vi "Control_Rack_Controler.vi"(0 "Times":dbl[](array[numeric]), 1 "Voltages Toroidal (Keep below |10|)":dbl[](array[numeric]), 2 "Voltages Helical (Keep below |10|)":dbl[](array[numeric]), 3 "error out":errorcluster, 4 "Data out 2":T2) -> (5 "error out 2":errorcluster, 6 "Data out":T2)   [LabVIEW 2017]
uses:
  Type_Defs/Data.ctl
  Type_Defs/Diagnostics.ctl
  Type_Defs/Systems.ctl
  <vilib>/DAQmx/write.llb/DAQmx Write (Analog DBL 1Chan 1Samp).vi
  <vilib>/DAQmx/create/channels.llb/DAQmx Create Channel (AO-Voltage-Basic).vi
  <vilib>/DAQmx/miscellaneous.llb/DAQmx Fill In Error Info.vi
  <vilib>/express/express shared/transition.llb/Dynamic To Waveform Array.vi
  <vilib>/express/express signal manip/GetorSetDDTAttributes/Set DDT Attributes/SetT0.vi
  <vilib>/express/express shared/transition.llb/Waveform Array To Dynamic.vi
  <vilib>/express/express signal manip/GetorSetDDTAttributes/Set DDT Attributes/Set DDT Properties.xnode
panel:
  out "Experiment State":T1(ring)
  out "Experiment Purpose":string
  out "Start Time":timestamp
  out "Experiment Number":i32
  out "Operator":string
  out "Running":bool
  out "hel_cur":dynamicdata(graph) caption="Helix Current Feedback"
  out "hel_vol":dynamicdata(graph) caption="Helix Voltage Feedback"
  out "hel_cur_set":dynamicdata(graph) caption="Helix Limited Current Set Point"
  out "torr_cur_set":dynamicdata(graph) caption="Torroidal Limited Current Set Point"
  out "torr_vol":dynamicdata(graph) caption="Torroidal Voltage Feedback"
  out "torr_cur":dynamicdata(graph) caption="Torroidal Current Feedback"
  out "Voltage Toroidal":dbl
  out "Time":dbl
  out "Voltage Helical":dbl
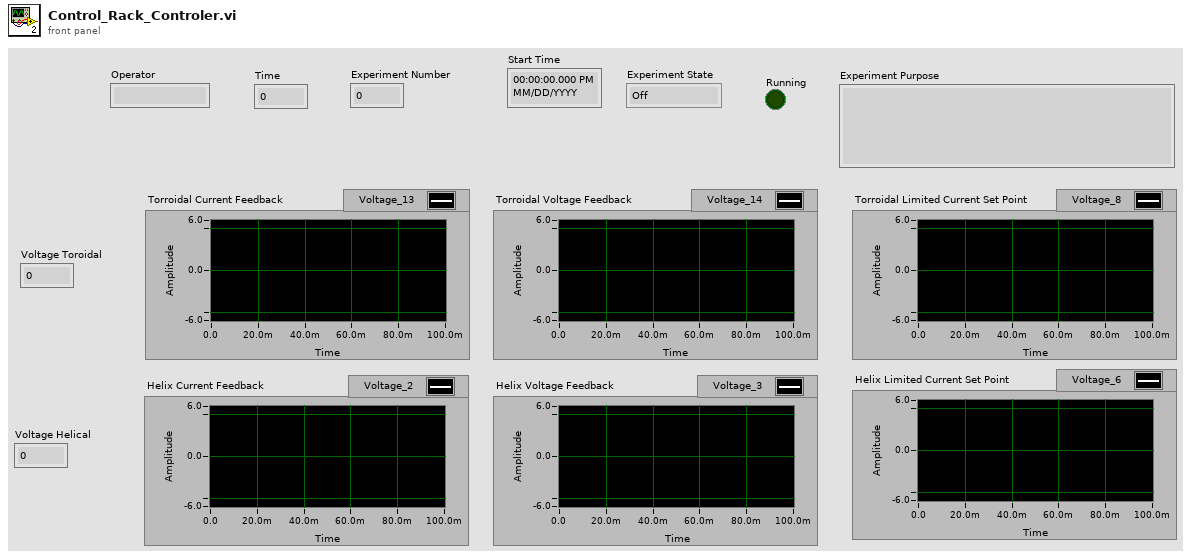
[diagram p1: front panel]
types:
  T1 = enum16{"Off", "Setting Up", "Ready", "In Progress", "Shutting Down"}
  T2 = typedef "Data.ctl" = cluster{"User Name":string, "Experiment Number":i32, "Start Time":timestamp, "Data":dbl[], "Step Number":i32, "Step Instructions":string, "Diagnostics":T3, "Experiment Purpose":string, "Experiment State":enum16{"Off", "Setting Up", "Ready", "In Progress", "Shutting Down"}, "Systems":T4, "Vacuum Pressure":dbl, "Fieldpoints":cluster{"System Boolean Fieldpoints":cluster{"Compressed Air":refnum<k21>, "T-20kV Power Switch":refnum<k21>, "T-Rectifier":refnum<k21>, "Engage Interlock":refnum<k21>, "Ventilator":refnum<k21>, "Magnetron":refnum<k21>, "H-20kV Power Switch":refnum<k21>, "H-Rectifier":refnum<k21>, "Main Water Pump":refnum<k21>, "WEGA Water Pump":refnum<k21>, "Gas Inlet Valves":refnum<k21>}, "Step Fieldpoints":cluster{"Exhaust Ventillator":refnum<k21>, "Compressed Air":refnum<k21>, "Water Pressure":refnum<k21>, "Interlock":refnum<k21>, "Toroidal Power Supply 1":refnum<k21>, "Toroidal Power Supply 2":refnum<k21>, "Toroidal Rectifier":refnum<k21>, "Helical Power Supply":refnum<k21>, "Helical Rectifier":refnum<k21>, "6kW Magnetron Standby":refnum<k21>, "20kW Magnetron Standby":refnum<k21>}}, "Pressure History":cluster{"Seconds into Experiment":i32[], "Pressure Data":dbl[]}, "Time Computer Control":dbl[], "Toroidal Voltage Computer Control":dbl[], "Helical Voltage Computer Control":dbl[], "Toroidal Current":dbl[], "Toroidal Voltage":dbl[], "Toroidal Current Set Point":dbl[], "Helical Current Set Point":dbl[], "Helical Voltage":dbl[], "Helical Current":dbl[], "Experiment Folder":path, "Run Another Shot?":bool}
  T3 = typedef "Diagnostics.ctl" = cluster{"Langmuir Probe":bool, "Rogowski 1":bool, "Rogowski 2":bool, "Rogowski 3":bool, "B-dot 1":bool, "B-dot 2":bool}
  T4 = typedef "Systems.ctl" = cluster{"Compressed Air":bool, "T-20kV Power Switch":bool, "T-Rectifier":bool, "Engage Interlock":bool, "Ventilator":bool, "Magnetron":bool, "H-20kV Power Switch":bool, "H-Rectifier":bool, "Main Water Pump":bool, "WEGA Water Pump":bool, "Gas Inlet Valves":bool}
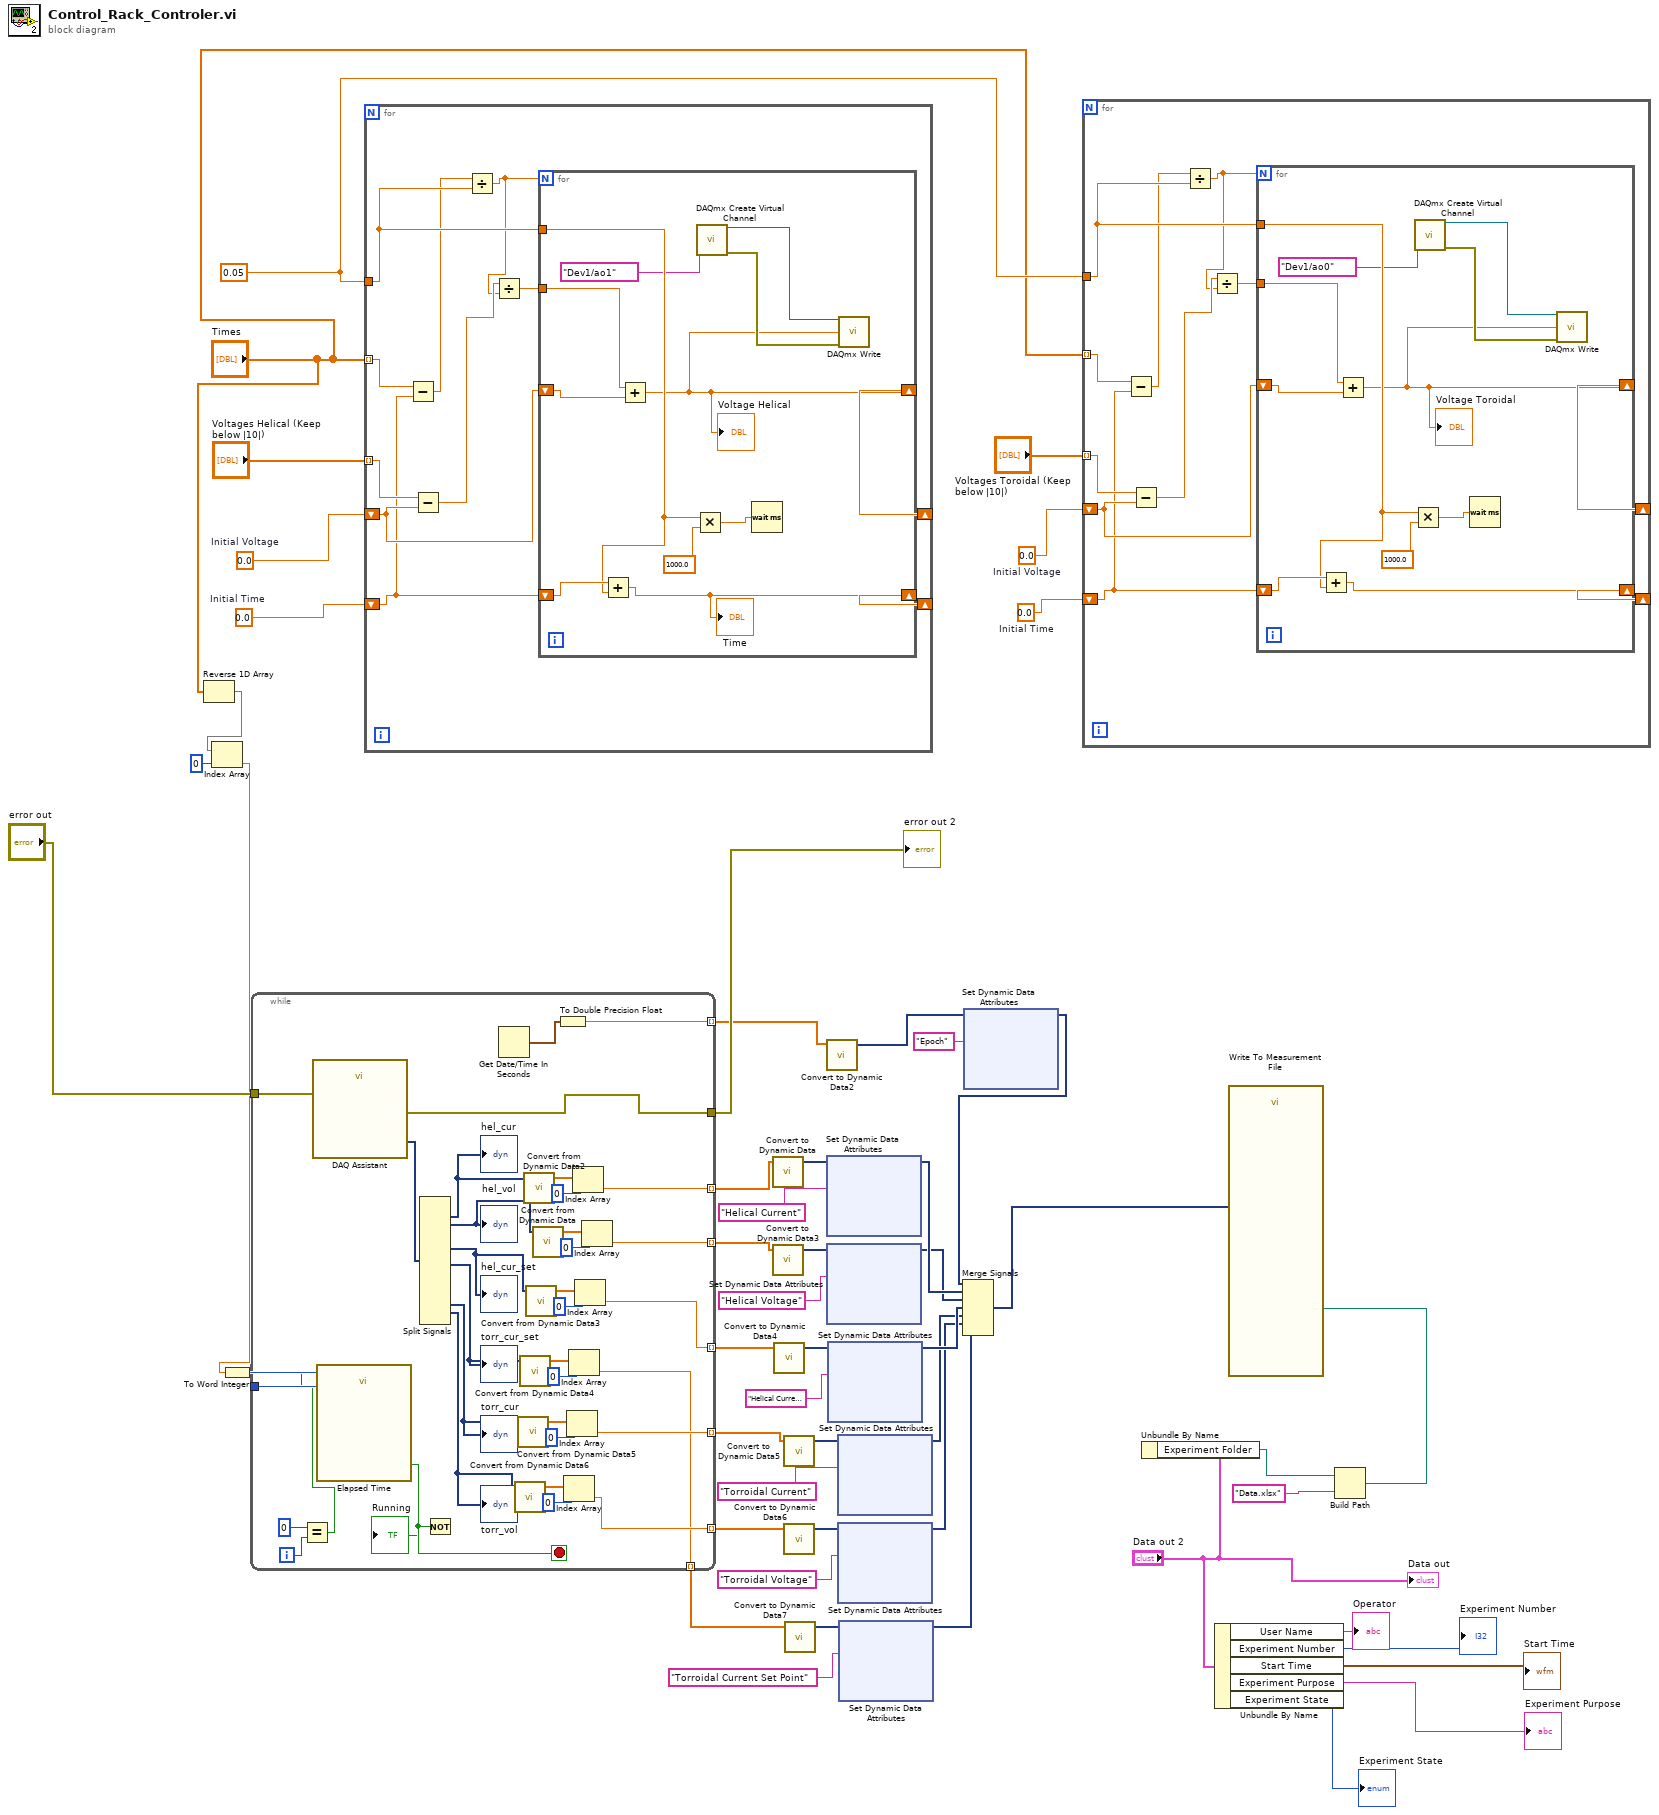
[diagram p0: block diagram]
diagram:
  w46 = 0.05 ("Timestep (in seconds, keep above 1/20s)")
  w49 = 0.0  # Initial Time
  w48 = 0.0  # Initial Voltage
  w50 = 0.0  # Initial Time
  w51 = 0.0  # Initial Voltage
  n1 = Reverse 1D Array(array="Times") -> (reversed array=w44:dbl[])
  n2 = Index Array(array=w44, index=0) -> (element=w40:dbl)
  n3 = To Word Integer(number=w40) -> (16bit integer=w39:i16)
  n4 = while {
    tunnel: "error out" -> [w86]
    tunnel: [w53] -> w41
    tunnel: w39 -> [w85]
    tunnel: [w56] -> w2 mode=indexing
    tunnel: [w66] -> w13 mode=indexing
    tunnel: [w55] -> w12 mode=indexing
    tunnel: [w65] -> w11 mode=indexing
    tunnel: [w64] -> w10 mode=indexing
    tunnel: [w63] -> w9 mode=indexing
    tunnel: [w57] -> w1 mode=indexing
    i -> [w54]
    stop <- w60 stop-if-true
    n5 = Equal?(x=0, y=w54) -> (x = y?=w61:bool)
    n6 = call "DAQ Assistant"("error in"=w86) -> ("data"=w87:dynamicdata, "error out"=w53:errorcluster)  [unwired: 16 in, 1 out]
    n7 = call "Elapsed Time"("Time Target (s)"=w85, "Reset"=w61) -> ("Time has Elapsed"=w60:bool)  [unwired: 10 in, 7 out]
    n8 = Split Signals(w87) -> (w84:dynamicdata, w71:dynamicdata, w70:dynamicdata, w69:dynamicdata, w68:dynamicdata, w67:dynamicdata)  [unwired: 16 in, 10 out]
    "hel_cur" <- w84
    "hel_vol" <- w71
    "hel_cur_set" <- w70
    "torr_cur_set" <- w69
    "torr_vol" <- w67
    "torr_cur" <- w68
    n9 = Not(x=w60) -> (.not. x?=→"Running":bool)
    n10 = Get Date/Time In Seconds() -> (seconds since 1Jan1904=w58:timestamp)
    n11 = call "Convert from Dynamic Data6"("Dynamic Data Type"=w67) -> ("Array"=w73:dbl[])  [unwired: 3 in]
    n12 = call "Convert from Dynamic Data5"("Dynamic Data Type"=w68) -> ("Array"=w75:dbl[])  [unwired: 3 in]
    n13 = call "Convert from Dynamic Data4"("Dynamic Data Type"=w69) -> ("Array"=w77:dbl[])  [unwired: 3 in]
    n14 = call "Convert from Dynamic Data2"("Dynamic Data Type"=w84) -> ("Array"=w83:dbl[])  [unwired: 3 in]
    n15 = call "Convert from Dynamic Data3"("Dynamic Data Type"=w70) -> ("Array"=w79:dbl[])  [unwired: 3 in]
    n16 = call "Convert from Dynamic Data"("Dynamic Data Type"=w71) -> ("Array"=w81:dbl[])  [unwired: 3 in]
    n17 = To Double Precision Float(number=w58) -> (double precision float=w57:dbl)
    n18 = Index Array(array=w73, index=0) -> (element=w64:dbl)
    n19 = Index Array(array=w75, index=0) -> (element=w65:dbl)
    n20 = Index Array(array=w77, index=0) -> (element=w63:dbl)
    n21 = Index Array(array=w83, index=0) -> (element=w56:dbl)
    n22 = Index Array(array=w79, index=0) -> (element=w55:dbl)
    n23 = Index Array(array=w81, index=0) -> (element=w66:dbl)
  }
  "error out 2" <- w41
  n24 = for {
    tunnel: "Voltages Helical (Keep below |10|)" -> [w98] mode=indexing
    tunnel: "Times" -> [w91] mode=indexing
    tunnel: w46 -> [w93]
    shift-right: [w94] -> _
    shift-left: w51 -> [w97]
    shift-right: [w92] -> _
    shift-left: w50 -> [w90]
    n25 = Subtract(x=w91, y=w90) -> (x-y=w89:dbl)
    n26 = Subtract(x=w98, y=w97) -> (x-y=w96:dbl)
    n27 = Divide(x=w89, y=w93) -> (x/y=w88:dbl)
    n28 = Divide(x=w96, y=w88) -> (x/y=w95:dbl)
    n29 = for {
      N: w88 -> [_]
      shift-right: [w99] -> w94
      shift-left: w97 -> [w109]
      tunnel: w95 -> [w108]
      tunnel: w93 -> [w105]
      shift-right: [w103] -> w92
      shift-left: w90 -> [w107]
      n30 = Add(x=w107, y=w105) -> (x+y=w103:dbl)
      "Time" <- w103
      n31 = Add(x=w108, y=w109) -> (x+y=w99:dbl)
      "Voltage Helical" <- w99
      n32 = Multiply(x=w105, y=1000.0) -> (x*y=w106:dbl)
      n33 = call-poly <vilib>:"DAQmx Create Virtual Channel.vi"("physical channels"=tag "Dev1/ao1" ("write channel (torr = ao0, hel = ao1)")) -> ("task out"=w100:refnum<k21>, "error out"=w101:errorcluster)  [unwired: 13 in]
      n34 = Wait (ms)(milliseconds to wait=w106) -> ()  [unwired: 1 out]
      n35 = call-poly <vilib>:"DAQmx Write.vi"("task/channels in"=w100, "data"=w99, "error in"=w101) -> ()  [unwired: 10 in, 3 out]
    }
  }
  n36 = call "Convert to Dynamic Data"("Array"=w2) -> ("Dynamic Data Type"=w35:dynamicdata)  [unwired: 3 in]
  n37 = call "Convert to Dynamic Data3"("Array"=w13) -> ("Dynamic Data Type"=w28:dynamicdata)  [unwired: 3 in]
  n38 = call "Convert to Dynamic Data4"("Array"=w12) -> ("Dynamic Data Type"=w27:dynamicdata)  [unwired: 3 in]
  n39 = call "Convert to Dynamic Data5"("Array"=w11) -> ("Dynamic Data Type"=w26:dynamicdata)  [unwired: 3 in]
  n40 = call "Convert to Dynamic Data6"("Array"=w10) -> ("Dynamic Data Type"=w24:dynamicdata)  [unwired: 3 in]
  n41 = call "Convert to Dynamic Data7"("Array"=w9) -> ("Dynamic Data Type"=w23:dynamicdata)  [unwired: 3 in]
  n42 = call "Convert to Dynamic Data2"("Array"=w1) -> ("Dynamic Data Type"=w33:dynamicdata)  [unwired: 3 in]
  n43 = xnode "Set Dynamic Data Attributes"("Signals In"=w35, "Signal Name"="Helical Current") -> ("Signals Out"=w31:dynamicdata)  [unwired: 2 in, 1 out]
  n44 = xnode "Set Dynamic Data Attributes"("Signals In"=w28, "Signal Name"="Helical Voltage") -> ("Signals Out"=w22:dynamicdata)  [unwired: 2 in, 1 out]
  n45 = xnode "Set Dynamic Data Attributes"("Signals In"=w27, "Signal Name"="Helical Current Set Point") -> ("Signals Out"=w21:dynamicdata)  [unwired: 2 in, 1 out]
  n46 = xnode "Set Dynamic Data Attributes"("Signals In"=w26, "Signal Name"="Torroidal Current") -> ("Signals Out"=w20:dynamicdata)  [unwired: 2 in, 1 out]
  n47 = xnode "Set Dynamic Data Attributes"("Signals In"=w24, "Signal Name"="Torroidal Voltage") -> ("Signals Out"=w19:dynamicdata)  [unwired: 2 in, 1 out]
  n48 = xnode "Set Dynamic Data Attributes"("Signals In"=w23, "Signal Name"="Torroidal Current Set Point") -> ("Signals Out"=w18:dynamicdata)  [unwired: 2 in, 1 out]
  n49 = xnode "Set Dynamic Data Attributes"("Signals In"=w33, "Signal Name"="Epoch") -> ("Signals Out"=w30:dynamicdata)  [unwired: 2 in, 1 out]
  n50 = Merge Signals(w30, w31, w22, w21, w20, w19, w18) -> (w29:dynamicdata)
  n51 = for {
    tunnel: "Voltages Toroidal (Keep below |10|)" -> [w120] mode=indexing
    tunnel: "Times" -> [w113] mode=indexing
    tunnel: w46 -> [w115]
    shift-right: [w116] -> _
    shift-left: w48 -> [w119]
    shift-right: [w114] -> _
    shift-left: w49 -> [w112]
    n52 = Subtract(x=w113, y=w112) -> (x-y=w111:dbl)
    n53 = Subtract(x=w120, y=w119) -> (x-y=w118:dbl)
    n54 = Divide(x=w111, y=w115) -> (x/y=w110:dbl)
    n55 = Divide(x=w118, y=w110) -> (x/y=w117:dbl)
    n56 = for {
      N: w110 -> [_]
      shift-right: [w121] -> w116
      shift-left: w119 -> [w131]
      tunnel: w117 -> [w130]
      tunnel: w115 -> [w127]
      shift-right: [w125] -> w114
      shift-left: w112 -> [w129]
      n57 = Add(x=w129, y=w127) -> (x+y=w125:dbl)
      n58 = Add(x=w130, y=w131) -> (x+y=w121:dbl)
      "Voltage Toroidal" <- w121
      n59 = Multiply(x=w127, y=1000.0) -> (x*y=w128:dbl)
      n60 = call-poly <vilib>:"DAQmx Create Virtual Channel.vi"("physical channels"=tag "Dev1/ao0" ("write channel (torr = ao0, hel = ao1) 2")) -> ("task out"=w122:refnum<k21>, "error out"=w123:errorcluster)  [unwired: 13 in]
      n61 = Wait (ms)(milliseconds to wait=w128) -> ()  [unwired: 1 out]
      n62 = call-poly <vilib>:"DAQmx Write.vi"("task/channels in"=w122, "data"=w121, "error in"=w123) -> ()  [unwired: 10 in, 3 out]
    }
  }
  n63 = Unbundle By Name("Data out 2") -> ("Experiment Folder"=w37:path)
  n64 = Unbundle By Name("Data out 2") -> ("User Name"=→"Operator":string, "Experiment Number"=→"Experiment Number":i32, "Start Time"=→"Start Time":timestamp, "Experiment Purpose"=→"Experiment Purpose":string, "Experiment State"=→"Experiment State":T1)
  n65 = Build Path(base path=w37, name or relative path="Data.xlsx") -> (appended path=w38:path)
  n66 = call "Write To Measurement File"("Signals"=w29, "Filename"=w38) -> ()  [unwired: 15 in, 3 out]
  "Data out" <- "Data out 2"
